vi "DAQ Test.vi"() -> ()   [LabVIEW 2015]
uses:
  <vilib>/DAQmx/read.llb/DAQmx Read (Analog 1D DBL 1Chan NSamp).vi
  <vilib>/Analysis/baseanly.llb/Mean (DBL).vi
  <vilib>/Analysis/2dsp.llb/Real FFT.vi
  <vilib>/DAQmx/create/channels.llb/DAQmx Create Channel (AI-Voltage-Basic).vi
  <vilib>/DAQmx/configure/timing.llb/DAQmx Timing (Sample Clock).vi
  <vilib>/DAQmx/miscellaneous.llb/DAQmx Fill In Error Info.vi
  <vilib>/Analysis/NI_AALPro.lvlib
  <vilib>/Analysis/NI_AALBase.lvlib
panel:
  out "mean":dbl format="%.5f"
  out "Integrated":dbl(graph)
  out "Integrated":dbl
  out "Frequency":dbl[](graph)
  out "Amplitude":dbl[](graph)
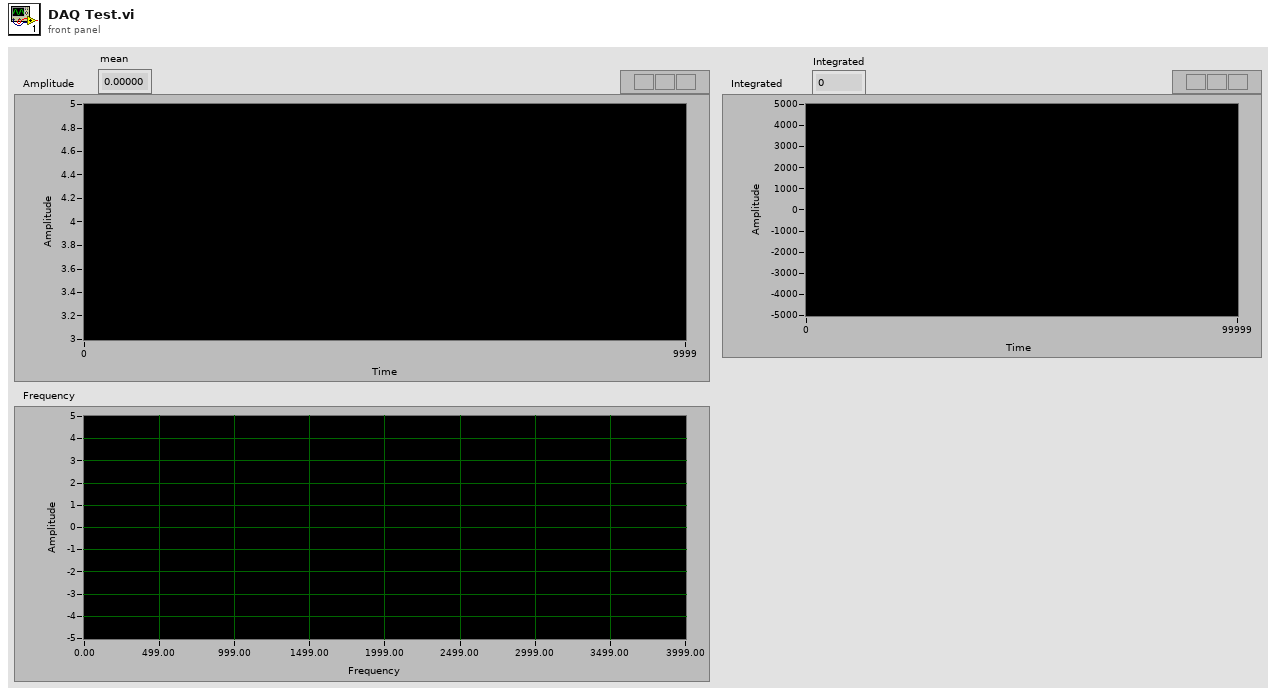
[diagram p1: front panel]
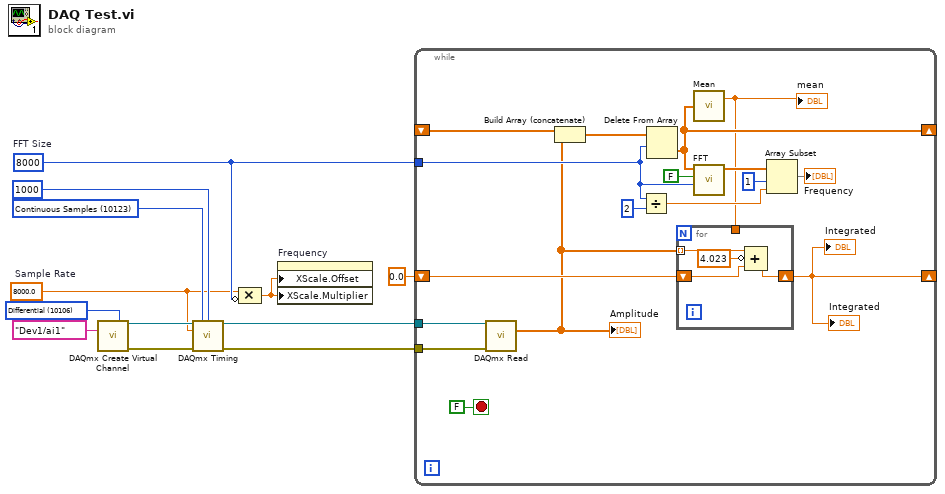
[diagram p0: block diagram]
diagram:
  w4 = 8000  # FFT Size
  w3 = 8000.0  # Sample Rate
  w6 = 10123 items=["Finite Samples"=10178, "Continuous Samples"=10123, "Hardware Timed Single Point"=12522] ("sample mode")
  w11 = 10106 items=["default"=-1, "RSE"=10083, "NRSE"=10078, "Differential"=10106, "Pseudodifferential"=12529] ("input terminal configuration")
  n1 = call-poly <vilib>:"DAQmx Create Virtual Channel.vi"("input terminal configuration"=w11, "physical channels"=tag "Dev1/ai1") -> ("task out"=w10:refnum<k21>, "error out"=w9:errorcluster)  [unwired: 12 in]
  n2 = call-poly <vilib>:"DAQmx Timing.vi"("task/channels in"=w10, "sample mode"=w6, "samples per channel"=1000, "rate"=w3, "error in"=w9) -> ("task out"=w8:refnum<k21>, "error out"=w7:errorcluster)  [unwired: 9 in]
  n3 = Compound Arithmetic op=MULTIPLY(w3, invert w4) -> (w2:dbl)
  n4 = property on="Frequency" class="WFGraph (strict)"("XScale.Offset"=w2, "XScale.Multiplier"=w2) -> ()  [unwired: 2 in, 2 out]
  n5 = while {
    tunnel: w8 -> [w29]
    tunnel: w7 -> [w28]
    shift-right: [w14] -> _
    shift-left: _ -> [w26]
    tunnel: w4 -> [w18]
    shift-right: [w16] -> _
    shift-left: 0.0 -> [w17]
    stop <- FALSE stop-if-true
    n6 = call-poly <vilib>:"DAQmx Read.vi"("task/channels in"=w29, "error in"=w28) -> ("data"=w15:dbl[])  [unwired: 11 in, 2 out]
    "Amplitude" <- w15
    n7 = Build Array (concatenate)(w26, w15) -> (w25:dbl[])
    n8 = Divide(x=w18, y=2) -> (x/y=w20:dbl)
    n9 = Delete From Array(array=w25, length=w18) -> (deleted portion=w14:dbl[])  [unwired: 1 in, 1 out]
    n10 = call-poly <vilib>:"Mean.vi"("X"=w14) -> ("mean"=w13:dbl)  [unwired: 1 out]
    "mean" <- w13
    n11 = for {
      tunnel: w15 -> [w33] mode=indexing
      shift-right: [w32] -> w16
      shift-left: w17 -> [w31]
      tunnel: w13 -> [_]
      n12 = Compound Arithmetic op=ADD(w33, invert 4.023 ("y"), w31) -> (w32:dbl)
    }
    "Integrated" <- w16
    "Integrated" <- w16
    n13 = call-poly <vilib>:"FFT.vi"("FFT size"=w18, "shift?"=FALSE, "X"=w14) -> ("FFT {X}"=w23:cdb[])  [unwired: 7 in, 1 out]
    n14 = Array Subset(array=w23, index=1, length=w20) -> (→"Frequency":cdb[])
  }
